vi "Updater Delete Old Clients.vi"(8 "error in (no error)":errorcluster) -> (0 "error out":errorcluster)   [LabVIEW 2011]
uses:
  OpenG.LIB/array/array.llb/Filter 1D Array (String)__ogtk.vi
  OpenG.LIB/file/file.llb/Build Path - File Names Array__ogtk.vi
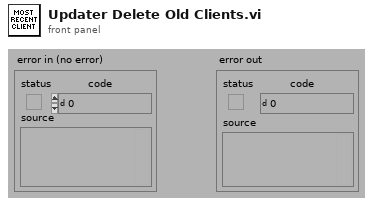
[diagram p1: front panel]
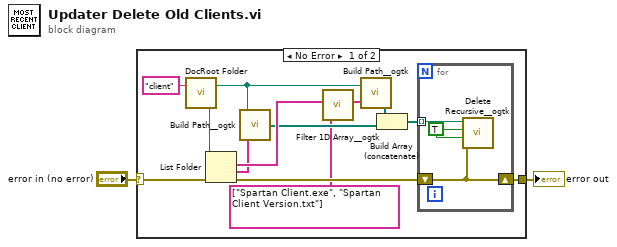
[diagram p0: block diagram]
diagram:
  n1 = case shown="No Error" "error in (no error)" {
    selector: "error in (no error)" -> [w3 w18]
    tunnel: [w12 w18] -> w1
    frame No Error {
      n2 = call "DocRoot Folder.vi"("Relative Path (\"\" - Folder)"="client" ("name or relative path")) -> ("DocumentRoot Folder"=w4:path)  [unwired: 2 in]
      n3 = List Folder(path=w4, error in=w3) -> (filenames=w14:string[], folder names=w11:string[], error out=w8:errorcluster)  [unwired: 2 in, 1 out]
      n4 = call-poly "Build Path__ogtk.vi"("name or relative path"=w11, "base path"=w4) -> ("appended path"=w10:path[])
      n5 = call-poly "Filter 1D Array__ogtk.vi"("items to filter"=string[] ["Spartan Client.exe", "Spartan Client Version.txt"], "array"=w14) -> ("filtered array"=w13:string[])  [unwired: 4 in, 1 out]
      n6 = call-poly "Build Path__ogtk.vi"("name or relative path"=w13, "base path"=w4) -> ("appended path"=w9:path[])
      n7 = Build Array (concatenate)(w9, w10) -> (w7:path[])
      n8 = for {
        tunnel: w7 -> [w17] mode=indexing
        shift-right: [w15] -> w12
        shift-left: w8 -> [w15]
        w16 = TRUE ("Recursive? (FALSE)")
        n9 = call "Delete Recursive__ogtk.vi"("error in (no error)"=w15, "Ignore Read-Only? (FALSE)"=w16, "Recursive? (FALSE)"=w16, "Path"=w17) -> ()  [unwired: 6 in, 2 out]
      }
    }
    frame Error {
    }
  }
  "error out" <- w1
